vi "Test Call Chain Failure Report.vi"(8 "error in (no error)":errorcluster) -> (0 "error out":errorcluster)   [LabVIEW 2013]
uses:
  classes/Test Suite/Test Suite.lvclass
  classes/Test Suite/Define Test Suite (SimpleText Report).vi
  classes/Test/Test.lvclass
panel:
  out "CALL CHAIN FAILURE OK":bool
  out "?":string
  out "element":string
  out "Test Report File Contents":string
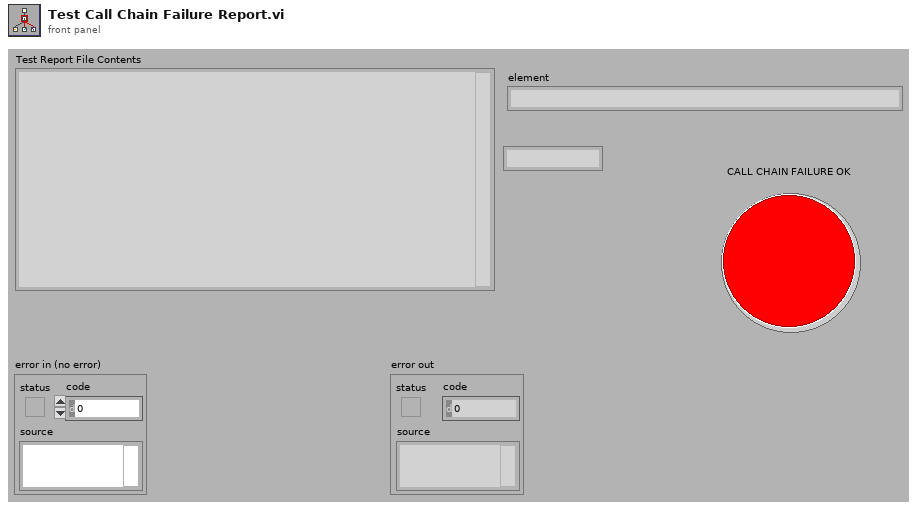
[diagram p1: front panel]
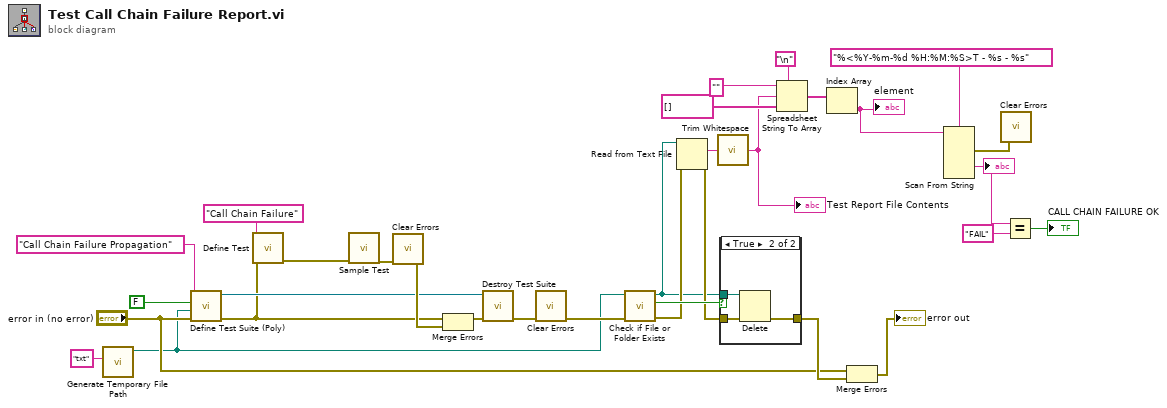
[diagram p0: block diagram]
diagram:
  n1 = call <vilib>:"Generate Temporary File Path.vi"("Temporary File Extension (tmp)"="txt") -> ("Unique Temporary File Path"=w13:path)  [unwired: 9 in, 1 out]
  n2 = call-poly "Define Test Suite (Poly).vi"("error in (no error)"="error in (no error)", "Report Path"=w13, "Interactive"=FALSE, "Label (VI Title)"="Call Chain Failure Propagation") -> ("error out"=w15:errorcluster, "Test Suite"=w17:refnum<class "Test Suite.lvclass">)  [unwired: 6 in]
  n3 = call "Define Test.vi"("error in (no error)"=w15, "Label (VI Title)"="Call Chain Failure") -> ("error out"=w24:errorcluster)  [unwired: 9 in]
  n4 = call "Sample Test.vi"("error in (no error)"=w24) -> ("error out"=w27:errorcluster)  [unwired: 10 in]
  n5 = call <vilib>:"Clear Errors.vi"("error in (no error)"=w27) -> ("error out"=w25:errorcluster)  [unwired: 6 in]
  n6 = Merge Errors(w15, w25) -> (w26:errorcluster)
  n7 = call-dynamic "Destroy Test Suite.vi"("error in (no error)"=w26, "Test Suite in"=w17) -> ("error out"=w22:errorcluster)  [unwired: 9 in]
  n8 = call <vilib>:"Clear Errors.vi"("error in (no error)"=w22) -> ("error out"=w21:errorcluster)  [unwired: 6 in]
  n9 = call <vilib>:"Check if File or Folder Exists.vi"("error in (no error)"=w21, "path"=w13) -> ("error out"=w30:errorcluster, "file or folder exists?"=w31:bool, "dup path"=w28:path)  [unwired: 7 in]
  n10 = Read from Text File(file (use dialog)=w28, error in=w30) -> (text=w12:string, error out=w29:errorcluster)  [unwired: 2 in, 2 out]
  n11 = call <vilib>:"Trim Whitespace.vi"("string"=w12) -> ("trimmed string"=w8:string)  [unwired: 1 in]
  "Test Report File Contents" <- w8
  n12 = case shown="True" w31 {
    tunnel: w28 -> [_ w36]
    tunnel: w29 -> [w33 w35]
    tunnel: [w33 w34] -> w19
    frame False {
    }
    frame True {
      n13 = Delete(path (use dialog)=w36, error in=w35) -> (error out=w34:errorcluster)  [unwired: 3 in, 2 out]
    }
  }
  n14 = Spreadsheet String To Array(delimiter (Tab)="\n", format string="", spreadsheet string=w8, array type (2D Dbl)=string[] []) -> (array=w7:string[])
  n15 = Index Array(array=w7) -> (element=w6:string)  [unwired: 1 in]
  "element" <- w6
  n16 = Merge Errors("error in (no error)", w19) -> (→"error out":errorcluster)
  n17 = Scan From String(format string="%<%Y-%m-%d %H:%M:%S>T - %s - %s", input string=w6) -> (error out=w1:errorcluster, output 2=w4:string)  [unwired: 7 in, 2 out]
  "?" <- w4
  n18 = call <vilib>:"Clear Errors.vi"("error in (no error)"=w1) -> ()  [unwired: 6 in, 1 out]
  n19 = Equal?(x=w4, y="FAIL") -> (x = y?=→"CALL CHAIN FAILURE OK":bool)
